vi "Fault_ID_Parse.vi"(8 "Enum":enum16{"Sequence", "Table"}(ring), 11 "Numeric":u32) -> (3 "String":string)   [LabVIEW 2016]
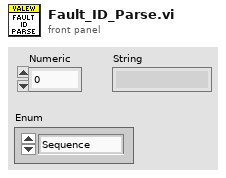
[diagram p1: front panel]
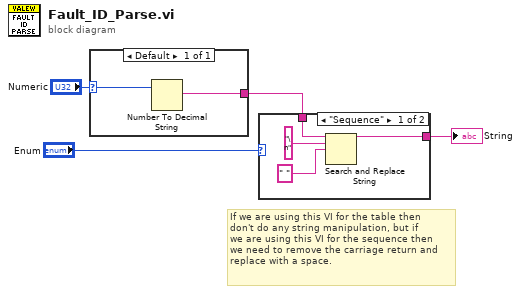
[diagram p0: block diagram]
diagram:
  # "If we are using this VI for the table then\ndon't do any string manipulation, but if\nwe are using this VI for the sequence then\nwe need to remove the carriage return and\nreplace with a space."
  n1 = case shown="Default" "Numeric" {
    selector: "Numeric" -> [w6]
    tunnel: [w5] -> w3
    frame Default {
      n2 = Number To Decimal String(number=w6) -> (decimal integer string=w5:string)  [unwired: 1 in]
    }
  }
  n3 = case shown="\"Sequence\"" "Enum" {
    tunnel: w3 -> [w10 w11]
    tunnel: [w7 w11] -> w2
    frame "Sequence" {
      n4 = Search and Replace String(input string=w10, search string="\n", replace string=" " ("replace string (\"\")")) -> (result string=w7:string)  [unwired: 5 in, 3 out]
    }
    frame "Table" {
    }
  }
  "String" <- w2
